vi "Run_Core.vi"(0 "Message Popup in":refnum<class "Array Functions.lvclass">, 11 "error in (no error)":errorcluster) -> (4 "Message Popup out":refnum<class "Array Functions.lvclass">, 6 "Return":variant, 15 "error out":errorcluster)   [LabVIEW 2019, in "Array Functions.lvclass"]
uses:
  Array Functions.lvclass
  C:/Users/Patrick/Documents/GitHub/LabVIEW-Script-Language/source code/LSL components/functions/functionsbase/functionbase.lvclass
  Array Functions.lvclass/Array Functions.ctl
  functionsbase/functionbase.lvclass/functionbase.ctl
  functionsbase/properties/Read RT Variables.vi
  functionsbase/properties/Read Indent#.vi
  data types/Variant to Data/Var to Numeric.vi
  data types/Variant to Data/Var to Boolean.vi
  variables/RT Variables/RT Variables.lvclass
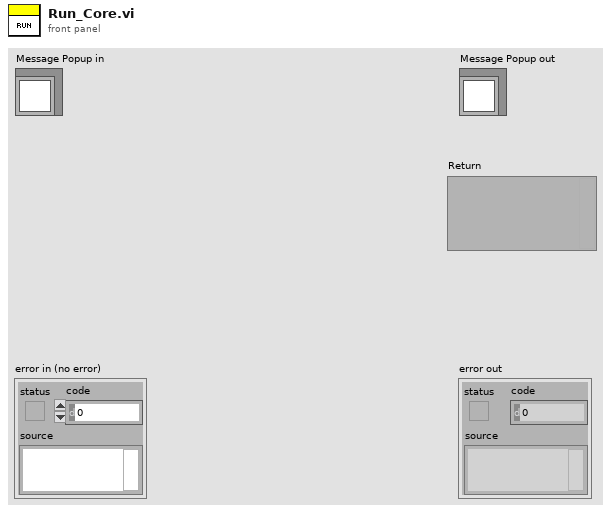
[diagram p1: front panel]
types:
  T1 = typedef "Array Functions.lvclass/Function List.ctl" = enum16{"Array Size", "Index Array", "Replace Subset", "Insert Into Array", "Delete From Array", "Initialize 1D Array", "Initialize 2D Array", "Build Array", "Array Subset", "Max in Array", "Min in Array", "Sort 1D Array", "Search 1D Aray", "Reverse 1D Array", "Slice by start stop", "Slice by start stop step", "range by start stop", "range by start stop step"}
  T2 = typedef "Datatype.ctl" = enum16{"Null", "Numeric", "String", "Bool", "Numeric 1D", "String 1D", "Bool 1D", "Numeric 2D", "String 2D", "Bool 2D", "Variant"}
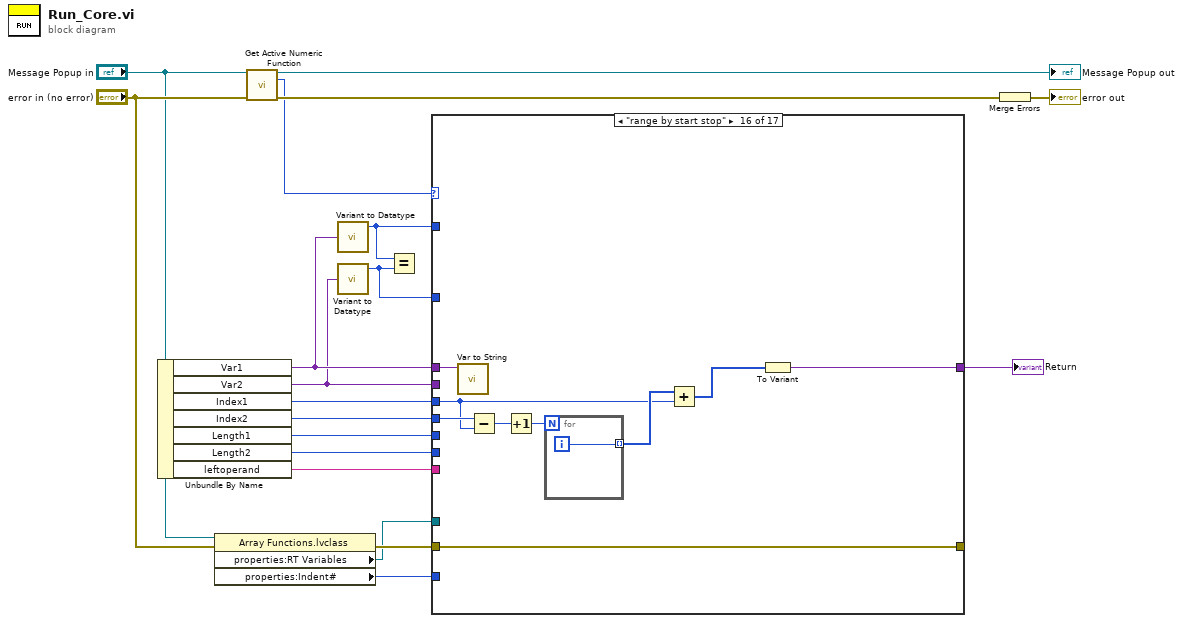
[diagram p0: block diagram]
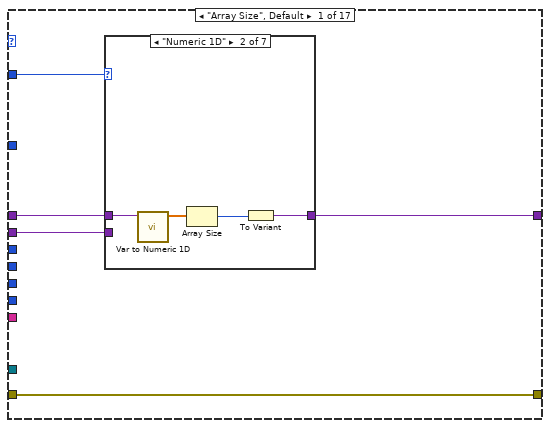
[diagram p2: hidden frame]
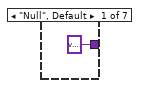
[diagram p3: hidden frame]
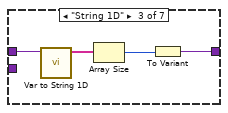
[diagram p4: hidden frame]
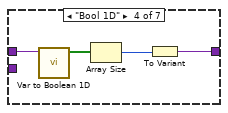
[diagram p5: hidden frame]
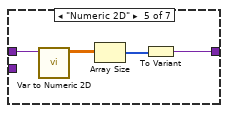
[diagram p6: hidden frame]
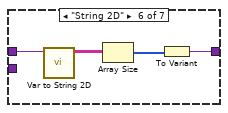
[diagram p7: hidden frame]
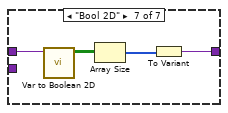
[diagram p8: hidden frame]
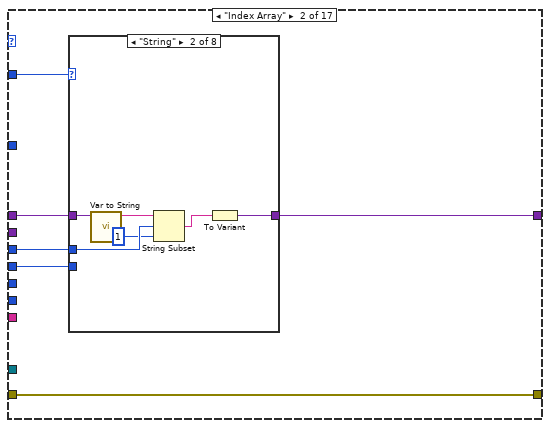
[diagram p9: hidden frame]
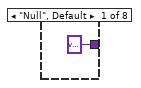
[diagram p10: hidden frame]
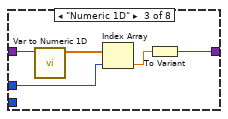
[diagram p11: hidden frame]
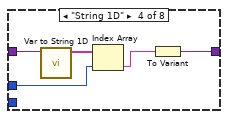
[diagram p12: hidden frame]
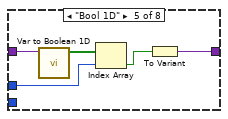
[diagram p13: hidden frame]
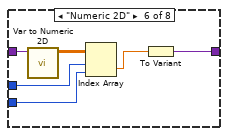
[diagram p14: hidden frame]
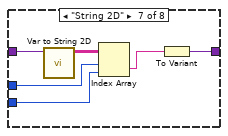
[diagram p15: hidden frame]
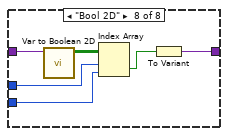
[diagram p16: hidden frame]
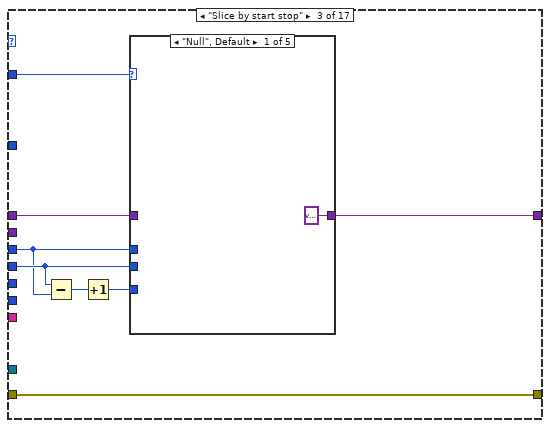
[diagram p17: hidden frame]
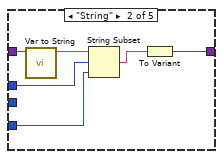
[diagram p18: hidden frame]
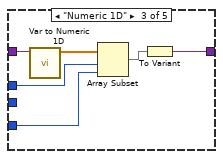
[diagram p19: hidden frame]
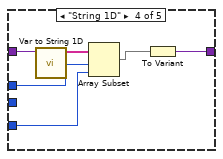
[diagram p20: hidden frame]
diagram:
  n1 = Unbundle By Name("Message Popup in") -> ("Var1"=w16:variant, "Var2"=w11:variant, "Index1"=w13:i32, "Index2"=w12:i32, "Length1"=w9:i32, "Length2"=w8:i32, "leftoperand"=w3:string)
  n2 = property class="Array Functions.lvclass"(reference="Message Popup in", error in="error in (no error)") -> (error out=w6:errorcluster, "properties:RT Variables"=w4:refnum<class "RT Variables.lvclass">, "properties:Indent#"=w2:i64)  [unwired: 1 out]
  n3 = call "Get Active Numeric Function.vi"("Numeric Functions in"="Message Popup in", "error in (no error)"="error in (no error)") -> ("Numeric Functions out"=→"Message Popup out":refnum<class "Array Functions.lvclass">, "Function"=w17:T1, "error out"=w18:errorcluster)  [unwired: 11 in]
  n4 = call "Variant to Datatype.vi"("Variant"=w16) -> ("Datatype"=w15:T2)  [unwired: 2 in, 2 out]
  n5 = call "Variant to Datatype.vi"("Variant"=w11) -> ("Datatype"=w10:T2)  [unwired: 2 in, 2 out]
  n6 = Equal?(x=w15, y=w10) -> ()  [unwired: 1 out]
  n7 = case shown="\"range by start stop\"" w17 {
    tunnel: w16 -> [w24 w55 w103 _ _ _ w319 w348 _ w493 w540 w568 _ w619 _ w671 w684]
    tunnel: w11 -> [w23 _ _ w140 w214 w289 _ _ w379 _ _ _ _ w617 _ _ _]
    tunnel: w15 -> [w22 w52 w101 _ _ _ w320 w345 _ w494 w541 w566 _ w618 _ _ _]
    tunnel: [w21 w54 w102 w131 w205 w278 w311 w338 w371 w490 w539 w567 w595 w615 w644 w670 w683] -> w14
    tunnel: w13 -> [_ w53 w98 w139 w213 w288 _ _ w378 w492 _ _ _ w616 _ w664 w679]
    tunnel: w12 -> [_ w51 w99 _ _ _ _ _ _ w489 _ _ _ _ _ w668 w681]
    tunnel: w10 -> [_ _ _ w141 w215 w290 _ _ w380 _ _ _ _ _ _ _ _]
    tunnel: w9 -> [_ _ _ _ _ w287 w318 w347 _ w491 _ _ _ _ _ _ w675]
    tunnel: w8 -> [_ _ _ _ _ _ _ w346 _ w488 _ _ _ _ _ _ _]
    tunnel: w6 -> [w20 w50 w100 w136 w210 w284 w317 w343 w375 w487 w538 w565 w599 w614 w648 w669 w682]
    tunnel: w4 -> [_ _ _ w135 w209 w281 w316 w342 w373 _ _ _ w598 _ w647 _ _]
    tunnel: w3 -> [_ _ _ w134 w206 w280 w312 w341 w372 _ _ _ w596 _ w645 _ _]
    tunnel: w2 -> [_ _ _ w132 w207 w282 w313 w339 w370 _ _ _ w597 _ w646 _ _]
    tunnel: [w20 w50 w100 w133 w208 w283 w310 w337 w374 w487 w538 w565 w594 w614 w643 w669 w682] -> _
    frame "Array Size", Default {
      n8 = case shown="\"Numeric 1D\"" w22 {
        tunnel: w24 -> [_ w29 w33 w37 w41 w45 w49]
        tunnel: w23 -> [_ _ _ _ _ _ _]
        tunnel: [variant ("Variant") w26 w30 w34 w38 w42 w46] -> w21
        frame "Null", Default {
        }
        frame "Numeric 1D" {
          n9 = call "Var to Numeric 1D.vi"("Variant"=w29) -> ("Numeric Array"=w28:dbl[])  [unwired: 10 in]
          n10 = Array Size(array=w28) -> (size(s)=w27:i32)
          n11 = To Variant(anything=w27) -> (Variant=w26:variant)
        }
        frame "String 1D" {
          n12 = call "Var to String 1D.vi"("Variant"=w33) -> ("String 1D"=w31:string[])  [unwired: 10 in]
          n13 = Array Size(array=w31) -> (size(s)=w32:i32)
          n14 = To Variant(anything=w32) -> (Variant=w30:variant)
        }
        frame "Bool 1D" {
          n15 = call "Var to Boolean 1D.vi"("Variant"=w37) -> ("Bool 1D"=w35:bool[])  [unwired: 10 in]
          n16 = Array Size(array=w35) -> (size(s)=w36:i32)
          n17 = To Variant(anything=w36) -> (Variant=w34:variant)
        }
        frame "Numeric 2D" {
          n18 = call "Var to Numeric 2D.vi"("Variant"=w41) -> ("Numeric Array"=w39:dbl[][])  [unwired: 10 in]
          n19 = Array Size(array=w39) -> (size(s)=w40:i32[])
          n20 = To Variant(anything=w40) -> (Variant=w38:variant)
        }
        frame "String 2D" {
          n21 = call "Var to String 2D.vi"("Variant"=w45) -> ("String 2D"=w43:string[][])  [unwired: 10 in]
          n22 = Array Size(array=w43) -> (size(s)=w44:i32[])
          n23 = To Variant(anything=w44) -> (Variant=w42:variant)
        }
        frame "Bool 2D" {
          n24 = call "Var to Boolean 2D.vi"("Variant"=w49) -> ("Bool 2D"=w47:bool[][])  [unwired: 10 in]
          n25 = Array Size(array=w47) -> (size(s)=w48:i32[])
          n26 = To Variant(anything=w48) -> (Variant=w46:variant)
        }
      }
    }
    frame "Index Array" {
      n27 = case shown="\"String\"" w52 {
        tunnel: w55 -> [_ w61 w67 w72 w77 w83 w89 w95]
        tunnel: [variant ("Variant") w62 w66 w71 w76 w82 w88 w94] -> w54
        tunnel: w53 -> [_ w59 w64 w68 w73 w79 w85 w91]
        tunnel: w51 -> [_ _ _ _ _ w78 w84 w90]
        frame "Null", Default {
        }
        frame "String" {
          n28 = call "Var to String.vi"("Variant"=w61) -> ("String"=w60:string)  [unwired: 10 in]
          n29 = String Subset(string=w60, offset (0)=w59, length (rest)=1 ("length (rest)")) -> (substring=w57:string)
          n30 = To Variant(anything=w57) -> (Variant=w62:variant)
        }
        frame "Numeric 1D" {
          n31 = call "Var to Numeric 1D.vi"("Variant"=w67) -> ("Numeric Array"=w65:dbl[])  [unwired: 10 in]
          n32 = Index Array(array=w65, index=w64) -> (element=w63:dbl)
          n33 = To Variant(anything=w63) -> (Variant=w66:variant)
        }
        frame "String 1D" {
          n34 = call "Var to String 1D.vi"("Variant"=w72) -> ("String 1D"=w70:string[])  [unwired: 10 in]
          n35 = Index Array(array=w70, index=w68) -> (element=w69:string)
          n36 = To Variant(anything=w69) -> (Variant=w71:variant)
        }
        frame "Bool 1D" {
          n37 = call "Var to Boolean 1D.vi"("Variant"=w77) -> ("Bool 1D"=w75:bool[])  [unwired: 10 in]
          n38 = Index Array(array=w75, index=w73) -> (element=w74:bool)
          n39 = To Variant(anything=w74) -> (Variant=w76:variant)
        }
        frame "Numeric 2D" {
          n40 = call "Var to Numeric 2D.vi"("Variant"=w83) -> ("Numeric Array"=w81:dbl[][])  [unwired: 10 in]
          n41 = Index Array(array=w81, index (row)=w79, index (col)=w78) -> (element=w80:dbl)
          n42 = To Variant(anything=w80) -> (Variant=w82:variant)
        }
        frame "String 2D" {
          n43 = call "Var to String 2D.vi"("Variant"=w89) -> ("String 2D"=w87:string[][])  [unwired: 10 in]
          n44 = Index Array(array=w87, index (row)=w85, index (col)=w84) -> (element=w86:string)
          n45 = To Variant(anything=w86) -> (Variant=w88:variant)
        }
        frame "Bool 2D" {
          n46 = call "Var to Boolean 2D.vi"("Variant"=w95) -> ("Bool 2D"=w93:bool[][])  [unwired: 10 in]
          n47 = Index Array(array=w93, index (row)=w91, index (col)=w90) -> (element=w92:bool)
          n48 = To Variant(anything=w92) -> (Variant=w94:variant)
        }
      }
    }
    frame "Slice by start stop" {
      n49 = Subtract(x=w99, y=w98) -> (x-y=w97:i32)
      n50 = Increment(x=w97) -> (x+1=w96:i32)
      n51 = case shown="\"Null\", Default" w101 {
        tunnel: w103 -> [_ w109 w116 w122 w128]
        tunnel: [variant ("Variant") w110 w115 w121 w127] -> w102
        tunnel: w98 -> [_ w106 w113 w118 w124]
        tunnel: w99 -> [_ _ _ _ _]
        tunnel: w96 -> [_ w105 w111 w117 w123]
        frame "Null", Default {
        }
        frame "String" {
          n52 = call "Var to String.vi"("Variant"=w109) -> ("String"=w108:string)  [unwired: 10 in]
          n53 = String Subset(string=w108, offset (0)=w106, length (rest)=w105) -> (substring=w107:string)
          n54 = To Variant(anything=w107) -> (Variant=w110:variant)
        }
        frame "Numeric 1D" {
          n55 = call "Var to Numeric 1D.vi"("Variant"=w116) -> ("Numeric Array"=w114:dbl[])  [unwired: 10 in]
          n56 = Array Subset(array=w114, index=w113, length=w111) -> (w112:dbl[])
          n57 = To Variant(anything=w112) -> (Variant=w115:variant)
        }
        frame "String 1D" {
          n58 = call "Var to String 1D.vi"("Variant"=w122) -> ("String 1D"=w120:string[])  [unwired: 10 in]
          n59 = Array Subset(array=w120, index=w118, length=w117) -> (w119:string[])
          n60 = To Variant(anything=w119) -> (Variant=w121:variant)
        }
        frame "Bool 1D" {
          n61 = call "Var to Boolean 1D.vi"("Variant"=w128) -> ("Bool 1D"=w126:bool[])  [unwired: 10 in]
          n62 = Array Subset(array=w126, index=w124, length=w123) -> (w125:bool[])
          n63 = To Variant(anything=w125) -> (Variant=w127:variant)
        }
      }
    }
    frame "Replace Subset" {
      n64 = call-dynamic "Retrieve RTV [by name].vi"("RT Variables in"=w135, "RTV name"=w134, "error in (no error)"=w136) -> ("RT Variables out"=w138:refnum<class "RT Variables.lvclass">, "Data"=w129:variant, "error out"=w137:errorcluster)  [unwired: 8 in, 2 out]
      n65 = call "Variant to Datatype.vi"("Variant"=w129) -> ("Datatype"=w130:T2)  [unwired: 2 in, 2 out]
      n66 = case shown="\"String 1D\"" w130 {
        tunnel: w129 -> [_ w147 w167 w187 _ _ _]
        tunnel: [variant ("Variant") w146 w163 w184 _ _ _] -> w131
        tunnel: w139 -> [_ w143 w164 w185 _ _ _]
        tunnel: w141 -> [_ w145 w166 w183 _ _ _]
        tunnel: w140 -> [_ w144 w165 w186 _ _ _]
        frame "Null", Default {
        }
        frame "Numeric 1D" {
          n67 = case shown="\"Numeric\"" w145 {
            tunnel: w147 -> [w151 w161 _]
            tunnel: [w150 w160 variant ("Variant")] -> w146
            tunnel: w144 -> [w149 w157 _]
            tunnel: w143 -> [w148 w156 _]
            frame "Numeric 1D" {
              n68 = call-poly "V2D_Poly.vi"("Variant"=w149) -> ("Numeric Array"=w152:dbl[])  [unwired: 10 in]
              n69 = call "Var to Numeric 1D.vi"("Variant"=w151) -> ("Numeric Array"=w154:dbl[])  [unwired: 10 in]
              n70 = Replace Array Subset(array=w154, new element=w152, index=w148) -> (w153:dbl[])
              n71 = To Variant(anything=w153) -> (Variant=w150:variant)
            }
            frame "Numeric" {
              n72 = call-poly "V2D_Poly.vi"("Variant"=w157) -> ("Numeric"=w155:dbl)  [unwired: 10 in]
              n73 = call "Var to Numeric 1D.vi"("Variant"=w161) -> ("Numeric Array"=w159:dbl[])  [unwired: 10 in]
              n74 = Replace Array Subset(array=w159, new element=w155, index=w156) -> (w158:dbl[])
              n75 = To Variant(anything=w158) -> (Variant=w160:variant)
            }
            frame Default {
            }
          }
        }
        frame "String 1D" {
          n76 = case shown="\"String 1D\"" w166 {
            tunnel: w167 -> [w171 w178 _]
            tunnel: [w172 w181 variant ("Variant")] -> w163
            tunnel: w165 -> [w169 w176 _]
            tunnel: w164 -> [w168 w175 _]
            frame "String 1D" {
              n77 = call-poly "V2D_Poly.vi"("Variant"=w171) -> ("String 1D"=w170:string[])  [unwired: 10 in]
              n78 = call-poly "V2D_Poly.vi"("Variant"=w169) -> ("String 1D"=w173:string[])  [unwired: 10 in]
              n79 = Replace Array Subset(array=w170, new element=w173, index=w168) -> (w174:string[])
              n80 = To Variant(anything=w174) -> (Variant=w172:variant)
            }
            frame "String" {
              n81 = call-poly "V2D_Poly.vi"("Variant"=w178) -> ("String 1D"=w177:string[])  [unwired: 10 in]
              n82 = call-poly "V2D_Poly.vi"("Variant"=w176) -> ("String"=w179:string)  [unwired: 10 in]
              n83 = Replace Array Subset(array=w177, new element=w179, index=w175) -> (w180:string[])
              n84 = To Variant(anything=w180) -> (Variant=w181:variant)
            }
            frame Default {
            }
          }
        }
        frame "Bool 1D" {
          n85 = case shown="\"Bool 1D\"" w183 {
            tunnel: w187 -> [w191 w198 _]
            tunnel: [w192 w201 variant ("Variant")] -> w184
            tunnel: w186 -> [w189 w196 _]
            tunnel: w185 -> [w188 w195 _]
            frame "Bool 1D" {
              n86 = call-poly "V2D_Poly.vi"("Variant"=w191) -> ("Bool 1D"=w190:bool[])  [unwired: 10 in]
              n87 = call-poly "V2D_Poly.vi"("Variant"=w189) -> ("Bool 1D"=w193:bool[])  [unwired: 10 in]
              n88 = Replace Array Subset(array=w190, new element=w193, index=w188) -> (w194:bool[])
              n89 = To Variant(anything=w194) -> (Variant=w192:variant)
            }
            frame "Bool" {
              n90 = call-poly "V2D_Poly.vi"("Variant"=w198) -> ("Bool 1D"=w197:bool[])  [unwired: 10 in]
              n91 = call-poly "V2D_Poly.vi"("Variant"=w196) -> ("Boolean"=w199:bool)  [unwired: 10 in]
              n92 = Replace Array Subset(array=w197, new element=w199, index=w195) -> (w200:bool[])
              n93 = To Variant(anything=w200) -> (Variant=w201:variant)
            }
            frame Default {
            }
          }
        }
        frame "Numeric 2D" {
        }
        frame "String 2D" {
        }
        frame "Bool 2D" {
        }
      }
      n94 = call-dynamic "Add RTV.vi"("RT Variables in"=w138, "RTV name"=w134, "Data"=w131, "Scope"=w132, "error in (no error)"=w137) -> ("error out"=w133:errorcluster)  [unwired: 9 in, 1 out]
    }
    frame "Insert Into Array" {
      n95 = call-dynamic "Retrieve RTV [by name].vi"("RT Variables in"=w209, "RTV name"=w206, "error in (no error)"=w210) -> ("RT Variables out"=w212:refnum<class "RT Variables.lvclass">, "Data"=w203:variant, "error out"=w211:errorcluster)  [unwired: 8 in, 2 out]
      n96 = call "Variant to Datatype.vi"("Variant"=w203) -> ("Datatype"=w204:T2)  [unwired: 2 in, 2 out]
      n97 = case shown="\"Numeric 1D\"" w204 {
        tunnel: w203 -> [_ w221 w241 w261 _ _ _]
        tunnel: [variant ("Variant") w220 w237 w258 _ _ _] -> w205
        tunnel: w213 -> [_ w217 w238 w259 _ _ _]
        tunnel: w215 -> [_ w219 w240 w257 _ _ _]
        tunnel: w214 -> [_ w218 w239 w260 _ _ _]
        frame "Null", Default {
        }
        frame "Numeric 1D" {
          n98 = case shown="\"Numeric\"" w219 {
            tunnel: w221 -> [w225 w235 _]
            tunnel: [w224 w234 variant ("Variant")] -> w220
            tunnel: w218 -> [w223 w231 _]
            tunnel: w217 -> [w222 w230 _]
            frame "Numeric 1D" {
              n99 = call-poly "V2D_Poly.vi"("Variant"=w223) -> ("Numeric Array"=w226:dbl[])  [unwired: 10 in]
              n100 = call "Var to Numeric 1D.vi"("Variant"=w225) -> ("Numeric Array"=w228:dbl[])  [unwired: 10 in]
              n101 = Insert Into Array(array=w228, index=w222, new element=w226) -> (w227:dbl[])
              n102 = To Variant(anything=w227) -> (Variant=w224:variant)
            }
            frame "Numeric" {
              n103 = call-poly "V2D_Poly.vi"("Variant"=w231) -> ("Numeric"=w229:dbl)  [unwired: 10 in]
              n104 = call "Var to Numeric 1D.vi"("Variant"=w235) -> ("Numeric Array"=w233:dbl[])  [unwired: 10 in]
              n105 = Insert Into Array(array=w233, index=w230, new element=w229) -> (w232:dbl[])
              n106 = To Variant(anything=w232) -> (Variant=w234:variant)
            }
            frame Default {
            }
          }
        }
        frame "String 1D" {
          n107 = case shown="\"String\"" w240 {
            tunnel: w241 -> [w245 w252 _]
            tunnel: [w246 w255 variant ("Variant")] -> w237
            tunnel: w239 -> [w243 w250 _]
            tunnel: w238 -> [w242 w249 _]
            frame "String 1D" {
              n108 = call-poly "V2D_Poly.vi"("Variant"=w245) -> ("String 1D"=w244:string[])  [unwired: 10 in]
              n109 = call-poly "V2D_Poly.vi"("Variant"=w243) -> ("String 1D"=w247:string[])  [unwired: 10 in]
              n110 = Insert Into Array(array=w244, index=w242, new element=w247) -> (w248:string[])
              n111 = To Variant(anything=w248) -> (Variant=w246:variant)
            }
            frame "String" {
              n112 = call-poly "V2D_Poly.vi"("Variant"=w252) -> ("String 1D"=w251:string[])  [unwired: 10 in]
              n113 = call-poly "V2D_Poly.vi"("Variant"=w250) -> ("String"=w253:string)  [unwired: 10 in]
              n114 = Insert Into Array(array=w251, index=w249, new element=w253) -> (w254:string[])
              n115 = To Variant(anything=w254) -> (Variant=w255:variant)
            }
            frame Default {
            }
          }
        }
        frame "Bool 1D" {
          n116 = case shown="\"Bool 1D\"" w257 {
            tunnel: w261 -> [w265 w272 _]
            tunnel: [w266 w275 variant ("Variant")] -> w258
            tunnel: w260 -> [w263 w270 _]
            tunnel: w259 -> [w262 w269 _]
            frame "Bool 1D" {
              n117 = call-poly "V2D_Poly.vi"("Variant"=w265) -> ("Bool 1D"=w264:bool[])  [unwired: 10 in]
              n118 = call-poly "V2D_Poly.vi"("Variant"=w263) -> ("Bool 1D"=w267:bool[])  [unwired: 10 in]
              n119 = Insert Into Array(array=w264, index=w262, new element=w267) -> (w268:bool[])
              n120 = To Variant(anything=w268) -> (Variant=w266:variant)
            }
            frame "Bool" {
              n121 = call-poly "V2D_Poly.vi"("Variant"=w272) -> ("Bool 1D"=w271:bool[])  [unwired: 10 in]
              n122 = call-poly "V2D_Poly.vi"("Variant"=w270) -> ("Boolean"=w273:bool)  [unwired: 10 in]
              n123 = Insert Into Array(array=w271, index=w269, new element=w273) -> (w274:bool[])
              n124 = To Variant(anything=w274) -> (Variant=w275:variant)
            }
            frame Default {
            }
          }
        }
        frame "Numeric 2D" {
        }
        frame "String 2D" {
        }
        frame "Bool 2D" {
        }
      }
      n125 = call-dynamic "Add RTV.vi"("RT Variables in"=w212, "RTV name"=w206, "Data"=w205, "Scope"=w207, "error in (no error)"=w211) -> ("error out"=w208:errorcluster)  [unwired: 9 in, 1 out]
    }
    frame "Delete From Array" {
      n126 = call-dynamic "Retrieve RTV [by name].vi"("RT Variables in"=w281, "RTV name"=w280, "error in (no error)"=w284) -> ("RT Variables out"=w286:refnum<class "RT Variables.lvclass">, "Data"=w277:variant, "error out"=w285:errorcluster)  [unwired: 8 in, 2 out]
      n127 = call "Variant to Datatype.vi"("Variant"=w277) -> ("Datatype"=w279:T2)  [unwired: 2 in, 2 out]
      n128 = case shown="\"String 1D\"" w279 {
        tunnel: w277 -> [_ w297 w303 w309 _ _ _]
        tunnel: [variant ("Variant") w296 w302 w308 _ _ _] -> w278
        tunnel: w288 -> [_ w293 w299 w305 _ _ _]
        tunnel: w290 -> [_ _ _ _ _ _ _]
        tunnel: w289 -> [_ _ _ _ _ _ _]
        tunnel: w287 -> [_ w292 w298 w304 _ _ _]
        frame "Null", Default {
        }
        frame "Numeric 1D" {
          n129 = call "Var to Numeric 1D.vi"("Variant"=w297) -> ("Numeric Array"=w295:dbl[])  [unwired: 10 in]
          n130 = Delete From Array(array=w295, length=w292, index=w293) -> (array with subset deleted=w294:dbl[])  [unwired: 1 out]
          n131 = To Variant(anything=w294) -> (Variant=w296:variant)
        }
        frame "String 1D" {
          n132 = call-poly "V2D_Poly.vi"("Variant"=w303) -> ("String 1D"=w300:string[])  [unwired: 10 in]
          n133 = Delete From Array(array=w300, length=w298, index=w299) -> (array with subset deleted=w301:string[])  [unwired: 1 out]
          n134 = To Variant(anything=w301) -> (Variant=w302:variant)
        }
        frame "Bool 1D" {
          n135 = call-poly "V2D_Poly.vi"("Variant"=w309) -> ("Bool 1D"=w306:bool[])  [unwired: 10 in]
          n136 = Delete From Array(array=w306, length=w304, index=w305) -> (array with subset deleted=w307:bool[])  [unwired: 1 out]
          n137 = To Variant(anything=w307) -> (Variant=w308:variant)
        }
        frame "Numeric 2D" {
        }
        frame "String 2D" {
        }
        frame "Bool 2D" {
        }
      }
      n138 = call-dynamic "Add RTV.vi"("RT Variables in"=w286, "RTV name"=w280, "Data"=w278, "Scope"=w282, "error in (no error)"=w285) -> ("error out"=w283:errorcluster)  [unwired: 9 in, 1 out]
    }
    frame "Initialize 1D Array" {
      n139 = call-dynamic "Retrieve RTV [by name].vi"("RT Variables in"=w316, "RTV name"=w312, "error in (no error)"=w317) -> ("RT Variables out"=w314:refnum<class "RT Variables.lvclass">, "error out"=w315:errorcluster)  [unwired: 8 in, 3 out]
      n140 = case shown="\"Numeric\"" w320 {
        tunnel: w319 -> [_ w324 w329 w336]
        tunnel: w318 -> [_ w322 w327 w334]
        tunnel: [variant ("Variant") w323 w328 w332] -> w311
        frame "Null", Default {
        }
        frame "Numeric" {
          n141 = call-poly "V2D_Poly.vi"("Variant"=w324) -> ("Numeric"=w326:dbl)  [unwired: 10 in]
          n142 = Initialize Array(w326, w322) -> (w325:dbl[])
          n143 = To Variant(anything=w325) -> (Variant=w323:variant)
        }
        frame "String" {
          n144 = call-poly "V2D_Poly.vi"("Variant"=w329) -> ("String"=w331:string)  [unwired: 10 in]
          n145 = Initialize Array(w331, w327) -> (w330:string[])
          n146 = To Variant(anything=w330) -> (Variant=w328:variant)
        }
        frame "Bool" {
          n147 = call-poly "V2D_Poly.vi"("Variant"=w336) -> ("Boolean"=w335:bool)  [unwired: 10 in]
          n148 = Initialize Array(w335, w334) -> (w333:bool[])
          n149 = To Variant(anything=w333) -> (Variant=w332:variant)
        }
      }
      n150 = call-dynamic "Add RTV.vi"("RT Variables in"=w314, "RTV name"=w312, "Data"=w311, "Scope"=w313, "error in (no error)"=w315) -> ("error out"=w310:errorcluster)  [unwired: 9 in, 1 out]
    }
    frame "Initialize 2D Array" {
      n151 = call-dynamic "Retrieve RTV [by name].vi"("RT Variables in"=w342, "RTV name"=w341, "error in (no error)"=w343) -> ("RT Variables out"=w344:refnum<class "RT Variables.lvclass">, "error out"=w340:errorcluster)  [unwired: 8 in, 3 out]
      n152 = case shown="\"String\"" w345 {
        tunnel: w348 -> [_ w353 w359 w367]
        tunnel: w347 -> [_ w351 w357 w365]
        tunnel: [variant ("Variant") w352 w358 w363] -> w338
        tunnel: w346 -> [_ w350 w356 w362]
        frame "Null", Default {
        }
        frame "Numeric" {
          n153 = call-poly "V2D_Poly.vi"("Variant"=w353) -> ("Numeric"=w355:dbl)  [unwired: 10 in]
          n154 = Initialize Array(w355, w351, w350) -> (w354:dbl[][])
          n155 = To Variant(anything=w354) -> (Variant=w352:variant)
        }
        frame "String" {
          n156 = call-poly "V2D_Poly.vi"("Variant"=w359) -> ("String"=w361:string)  [unwired: 10 in]
          n157 = Initialize Array(w361, w357, w356) -> (w360:string[][])
          n158 = To Variant(anything=w360) -> (Variant=w358:variant)
        }
        frame "Bool" {
          n159 = call-poly "V2D_Poly.vi"("Variant"=w367) -> ("Boolean"=w366:bool)  [unwired: 10 in]
          n160 = Initialize Array(w366, w365, w362) -> (w364:bool[][])
          n161 = To Variant(anything=w364) -> (Variant=w363:variant)
        }
      }
      n162 = call-dynamic "Add RTV.vi"("RT Variables in"=w344, "RTV name"=w341, "Data"=w338, "Scope"=w339, "error in (no error)"=w340) -> ("error out"=w337:errorcluster)  [unwired: 9 in, 1 out]
    }
    frame "Build Array" {
      # "append"
      n163 = call-dynamic "Retrieve RTV [by name].vi"("RT Variables in"=w373, "RTV name"=w372, "error in (no error)"=w375) -> ("RT Variables out"=w377:refnum<class "RT Variables.lvclass">, "Data"=w368:variant, "error out"=w376:errorcluster)  [unwired: 8 in, 2 out]
      n164 = call "Variant to Datatype.vi"("Variant"=w368) -> ("Datatype"=w369:T2)  [unwired: 2 in, 2 out]
      n165 = case shown="\"String 1D\"" w369 {
        tunnel: w368 -> [_ w386 w404 w422 w439 w456 w473]
        tunnel: [variant ("Variant") w385 w400 w419 w437 w453 w470] -> w371
        tunnel: w378 -> [_ w382 w401 w420 _ _ _]
        tunnel: w380 -> [_ w384 w403 w418 w436 w454 w471]
        tunnel: w379 -> [_ w383 w402 w421 w438 w455 w472]
        frame "Null", Default {
        }
        frame "Numeric 1D" {
          n166 = case shown="Default" w384 {
            tunnel: w386 -> [w389 w398 _]
            tunnel: [w388 w397 variant ("Variant")] -> w385
            tunnel: w383 -> [w387 w394 _]
            tunnel: w382 -> [_ _ _]
            frame "Numeric 1D" {
              n167 = call-poly "V2D_Poly.vi"("Variant"=w387) -> ("Numeric Array"=w390:dbl[])  [unwired: 10 in]
              n168 = call "Var to Numeric 1D.vi"("Variant"=w389) -> ("Numeric Array"=w392:dbl[])  [unwired: 10 in]
              n169 = Build Array (concatenate)(w392, w390) -> (w391:dbl[])
              n170 = To Variant(anything=w391) -> (Variant=w388:variant)
            }
            frame "Numeric" {
              n171 = call-poly "V2D_Poly.vi"("Variant"=w394) -> ("Numeric"=w393:dbl)  [unwired: 10 in]
              n172 = call "Var to Numeric 1D.vi"("Variant"=w398) -> ("Numeric Array"=w396:dbl[])  [unwired: 10 in]
              n173 = Build Array (concatenate)(w396, w393) -> (w395:dbl[])
              n174 = To Variant(anything=w395) -> (Variant=w397:variant)
            }
            frame Default {
            }
          }
        }
        frame "String 1D" {
          n175 = case shown="Default" w403 {
            tunnel: w404 -> [w407 w413 _]
            tunnel: [w408 w416 variant ("Variant")] -> w400
            tunnel: w402 -> [w405 w411 _]
            tunnel: w401 -> [_ _ _]
            frame "String 1D" {
              n176 = call-poly "V2D_Poly.vi"("Variant"=w407) -> ("String 1D"=w406:string[])  [unwired: 10 in]
              n177 = call-poly "V2D_Poly.vi"("Variant"=w405) -> ("String 1D"=w409:string[])  [unwired: 10 in]
              n178 = Build Array (concatenate)(w406, w409) -> (w410:string[])
              n179 = To Variant(anything=w410) -> (Variant=w408:variant)
            }
            frame "String" {
              n180 = call-poly "V2D_Poly.vi"("Variant"=w413) -> ("String 1D"=w412:string[])  [unwired: 10 in]
              n181 = call-poly "V2D_Poly.vi"("Variant"=w411) -> ("String"=w414:string)  [unwired: 10 in]
              n182 = Build Array (concatenate)(w412, w414) -> (w415:string[])
              n183 = To Variant(anything=w415) -> (Variant=w416:variant)
            }
            frame Default {
            }
          }
        }
        frame "Bool 1D" {
          n184 = case shown="\"Bool\"" w418 {
            tunnel: w422 -> [w425 w431 _]
            tunnel: [w426 w434 variant ("Variant")] -> w419
            tunnel: w421 -> [w423 w429 _]
            tunnel: w420 -> [_ _ _]
            frame "Bool 1D" {
              n185 = call-poly "V2D_Poly.vi"("Variant"=w425) -> ("Bool 1D"=w424:bool[])  [unwired: 10 in]
              n186 = call-poly "V2D_Poly.vi"("Variant"=w423) -> ("Bool 1D"=w427:bool[])  [unwired: 10 in]
              n187 = Build Array (concatenate)(w424, w427) -> (w428:bool[])
              n188 = To Variant(anything=w428) -> (Variant=w426:variant)
            }
            frame "Bool" {
              n189 = call-poly "V2D_Poly.vi"("Variant"=w431) -> ("Bool 1D"=w430:bool[])  [unwired: 10 in]
              n190 = call-poly "V2D_Poly.vi"("Variant"=w429) -> ("Boolean"=w432:bool)  [unwired: 10 in]
              n191 = Build Array (concatenate)(w430, w432) -> (w433:bool[])
              n192 = To Variant(anything=w433) -> (Variant=w434:variant)
            }
            frame Default {
            }
          }
        }
        frame "Numeric 2D" {
          n193 = case shown="\"Numeric 2D\"" w436 {
            tunnel: w439 -> [w441 w447 _]
            tunnel: [w443 w451 variant ("Variant")] -> w437
            tunnel: w438 -> [w442 w449 _]
            frame "Numeric 1D" {
              n194 = call-poly "V2D_Poly.vi"("Variant"=w442) -> ("Numeric Array"=w444:dbl[])  [unwired: 10 in]
              n195 = call-poly "V2D_Poly.vi"("Variant"=w441) -> ("Numeric Array"=w440:dbl[][])  [unwired: 10 in]
              n196 = Build Array (concatenate)(w440, w444) -> (w445:dbl[][])
              n197 = To Variant(anything=w445) -> (Variant=w443:variant)
            }
            frame "Numeric 2D" {
              n198 = call-poly "V2D_Poly.vi"("Variant"=w447) -> ("Numeric Array"=w446:dbl[][])  [unwired: 10 in]
              n199 = call-poly "V2D_Poly.vi"("Variant"=w449) -> ("Numeric Array"=w448:dbl[][])  [unwired: 10 in]
              n200 = Build Array (concatenate)(w446, w448) -> (w450:dbl[][])
              n201 = To Variant(anything=w450) -> (Variant=w451:variant)
            }
            frame Default {
            }
          }
        }
        frame "String 2D" {
          n202 = case shown="\"String 2D\"" w454 {
            tunnel: w456 -> [w459 w465 _]
            tunnel: [w460 w468 variant ("Variant")] -> w453
            tunnel: w455 -> [w457 w463 _]
            frame "String 1D" {
              n203 = call-poly "V2D_Poly.vi"("Variant"=w459) -> ("String 2D"=w458:string[][])  [unwired: 10 in]
              n204 = call-poly "V2D_Poly.vi"("Variant"=w457) -> ("String 1D"=w461:string[])  [unwired: 10 in]
              n205 = Build Array (concatenate)(w458, w461) -> (w462:string[][])
              n206 = To Variant(anything=w462) -> (Variant=w460:variant)
            }
            frame "String 2D" {
              n207 = call-poly "V2D_Poly.vi"("Variant"=w465) -> ("String 2D"=w464:string[][])  [unwired: 10 in]
              n208 = call-poly "V2D_Poly.vi"("Variant"=w463) -> ("String 2D"=w466:string[][])  [unwired: 10 in]
              n209 = Build Array (concatenate)(w464, w466) -> (w467:string[][])
              n210 = To Variant(anything=w467) -> (Variant=w468:variant)
            }
            frame Default {
            }
          }
        }
        frame "Bool 2D" {
          n211 = case shown="Default" w471 {
            tunnel: w473 -> [w476 w482 _]
            tunnel: [w477 w485 variant ("Variant")] -> w470
            tunnel: w472 -> [w474 w480 _]
            frame "Bool 1D" {
              n212 = call-poly "V2D_Poly.vi"("Variant"=w476) -> ("Bool 2D"=w475:bool[][])  [unwired: 10 in]
              n213 = call-poly "V2D_Poly.vi"("Variant"=w474) -> ("Bool 1D"=w478:bool[])  [unwired: 10 in]
              n214 = Build Array (concatenate)(w475, w478) -> (w479:bool[][])
              n215 = To Variant(anything=w479) -> (Variant=w477:variant)
            }
            frame "Bool 2D" {
              n216 = call-poly "V2D_Poly.vi"("Variant"=w482) -> ("Bool 2D"=w481:bool[][])  [unwired: 10 in]
              n217 = call-poly "V2D_Poly.vi"("Variant"=w480) -> ("Bool 2D"=w483:bool[][])  [unwired: 10 in]
              n218 = Build Array (concatenate)(w481, w483) -> (w484:bool[][])
              n219 = To Variant(anything=w484) -> (Variant=w485:variant)
            }
            frame Default {
            }
          }
        }
      }
      n220 = call-dynamic "Add RTV.vi"("RT Variables in"=w377, "RTV name"=w372, "Data"=w371, "Scope"=w370, "error in (no error)"=w376) -> ("error out"=w374:errorcluster)  [unwired: 9 in, 1 out]
    }
    frame "Array Subset" {
      n221 = case shown="\"Bool 1D\"" w494 {
        tunnel: w493 -> [_ w501 w505 w512 w520 w528 w536]
        tunnel: w492 -> [_ w499 w503 w511 w518 w526 w534]
        tunnel: w491 -> [_ w498 w502 w510 w517 w525 w533]
        tunnel: [variant ("Variant") w496 w504 w508 w514 w522 w530] -> w490
        tunnel: w489 -> [_ _ _ _ w516 w524 w532]
        tunnel: w488 -> [_ _ _ _ w515 w523 w531]
        frame "Null", Default {
        }
        frame "Numeric 1D" {
          n222 = call-poly "V2D_Poly.vi"("Variant"=w501) -> ("Numeric Array"=w500:dbl[])  [unwired: 10 in]
          n223 = Array Subset(array=w500, index=w499, length=w498) -> (w497:dbl[])
          n224 = To Variant(anything=w497) -> (Variant=w496:variant)
        }
        frame "String 1D" {
          n225 = call-poly "V2D_Poly.vi"("Variant"=w505) -> ("String 1D"=w507:string[])  [unwired: 10 in]
          n226 = Array Subset(array=w507, index=w503, length=w502) -> (w506:string[])
          n227 = To Variant(anything=w506) -> (Variant=w504:variant)
        }
        frame "Bool 1D" {
          n228 = call-poly "V2D_Poly.vi"("Variant"=w512) -> ("Bool 1D"=w513:bool[])  [unwired: 10 in]
          n229 = Array Subset(array=w513, index=w511, length=w510) -> (w509:bool[])
          n230 = To Variant(anything=w509) -> (Variant=w508:variant)
        }
        frame "Numeric 2D" {
          n231 = call-poly "V2D_Poly.vi"("Variant"=w520) -> ("Numeric Array"=w521:dbl[][])  [unwired: 10 in]
          n232 = Array Subset(array=w521, index (row)=w518, length (row)=w517, index (col)=w516, length (col)=w515) -> (w519:dbl[][])
          n233 = To Variant(anything=w519) -> (Variant=w514:variant)
        }
        frame "String 2D" {
          n234 = call-poly "V2D_Poly.vi"("Variant"=w528) -> ("String 2D"=w529:string[][])  [unwired: 10 in]
          n235 = Array Subset(array=w529, index (row)=w526, length (row)=w525, index (col)=w524, length (col)=w523) -> (w527:string[][])
          n236 = To Variant(anything=w527) -> (Variant=w522:variant)
        }
        frame "Bool 2D" {
          n237 = call-poly "V2D_Poly.vi"("Variant"=w536) -> ("Bool 2D"=w537:bool[][])  [unwired: 10 in]
          n238 = Array Subset(array=w537, index (row)=w534, length (row)=w533, index (col)=w532, length (col)=w531) -> (w535:bool[][])
          n239 = To Variant(anything=w535) -> (Variant=w530:variant)
        }
      }
    }
    frame "Max in Array" {
      n240 = case shown="\"Numeric 2D\"" w541 {
        tunnel: w540 -> [_ _ _ _ w549 w551 _ w556 w560 _ _]
        tunnel: [variant ("Variant") variant ("Variant") variant ("Variant") variant ("Variant") w546 w550 variant ("Variant") w555 w559 variant ("Variant") variant ("Variant")] -> w539
        frame "Null", Default {
        }
        frame "Numeric" {
        }
        frame "String" {
        }
        frame "Bool" {
        }
        frame "Numeric 1D" {
          n241 = call-poly "V2D_Poly.vi"("Variant"=w549) -> ("Numeric Array"=w548:dbl[])  [unwired: 10 in]
          n242 = Array Max & Min(array=w548) -> (max value=w547:dbl)  [unwired: 3 out]
          n243 = To Variant(anything=w547) -> (Variant=w546:variant)
        }
        frame "String 1D" {
          n244 = call-poly "V2D_Poly.vi"("Variant"=w551) -> ("String 1D"=w553:string[])  [unwired: 10 in]
          n245 = Array Max & Min(array=w553) -> (max value=w552:string)  [unwired: 3 out]
          n246 = To Variant(anything=w552) -> (Variant=w550:variant)
        }
        frame "Bool 1D" {
        }
        frame "Numeric 2D" {
          n247 = call-poly "V2D_Poly.vi"("Variant"=w556) -> ("Numeric Array"=w558:dbl[][])  [unwired: 10 in]
          n248 = Array Max & Min(array=w558) -> (max value=w557:dbl)  [unwired: 3 out]
          n249 = To Variant(anything=w557) -> (Variant=w555:variant)
        }
        frame "String 2D" {
          n250 = call-poly "V2D_Poly.vi"("Variant"=w560) -> ("String 2D"=w562:string[][])  [unwired: 10 in]
          n251 = Array Max & Min(array=w562) -> (max value=w561:string)  [unwired: 3 out]
          n252 = To Variant(anything=w561) -> (Variant=w559:variant)
        }
        frame "Bool 2D" {
        }
        frame "Variant" {
        }
      }
    }
    frame "Min in Array" {
      n253 = case shown="\"String 1D\"" w566 {
        tunnel: w568 -> [_ _ _ _ w576 w579 _ w584 w588 _ _]
        tunnel: [variant ("Variant") variant ("Variant") variant ("Variant") variant ("Variant") w574 w578 variant ("Variant") w583 w587 variant ("Variant") variant ("Variant")] -> w567
        frame "Null", Default {
        }
        frame "Numeric" {
        }
        frame "String" {
        }
        frame "Bool" {
        }
        frame "Numeric 1D" {
          n254 = call-poly "V2D_Poly.vi"("Variant"=w576) -> ("Numeric Array"=w575:dbl[])  [unwired: 10 in]
          n255 = Array Max & Min(array=w575) -> (min value=w573:dbl)  [unwired: 3 out]
          n256 = To Variant(anything=w573) -> (Variant=w574:variant)
        }
        frame "String 1D" {
          n257 = call-poly "V2D_Poly.vi"("Variant"=w579) -> ("String 1D"=w580:string[])  [unwired: 10 in]
          n258 = Array Max & Min(array=w580) -> (min value=w577:string)  [unwired: 3 out]
          n259 = To Variant(anything=w577) -> (Variant=w578:variant)
        }
        frame "Bool 1D" {
        }
        frame "Numeric 2D" {
          n260 = call-poly "V2D_Poly.vi"("Variant"=w584) -> ("Numeric Array"=w585:dbl[][])  [unwired: 10 in]
          n261 = Array Max & Min(array=w585) -> (min value=w582:dbl)  [unwired: 3 out]
          n262 = To Variant(anything=w582) -> (Variant=w583:variant)
        }
        frame "String 2D" {
          n263 = call-poly "V2D_Poly.vi"("Variant"=w588) -> ("String 2D"=w589:string[][])  [unwired: 10 in]
          n264 = Array Max & Min(array=w589) -> (min value=w586:string)  [unwired: 3 out]
          n265 = To Variant(anything=w586) -> (Variant=w587:variant)
        }
        frame "Bool 2D" {
        }
        frame "Variant" {
        }
      }
    }
    frame "Sort 1D Array" {
      n266 = call-dynamic "Retrieve RTV [by name].vi"("RT Variables in"=w598, "RTV name"=w596, "error in (no error)"=w599) -> ("RT Variables out"=w601:refnum<class "RT Variables.lvclass">, "Data"=w592:variant, "error out"=w600:errorcluster)  [unwired: 8 in, 2 out]
      n267 = call "Variant to Datatype.vi"("Variant"=w592) -> ("Datatype"=w593:T2)  [unwired: 2 in, 2 out]
      n268 = case shown="\"Numeric 1D\"" w593 {
        tunnel: w592 -> [_ w605 w607 w611]
        tunnel: [_ w602 w606 w610] -> w595
        frame "Null", Default {
        }
        frame "Numeric 1D" {
          n269 = call-poly "V2D_Poly.vi"("Variant"=w605) -> ("Numeric Array"=w604:dbl[])  [unwired: 10 in]
          n270 = Sort 1D Array(array=w604) -> (sorted array=w603:dbl[])
          n271 = To Variant(anything=w603) -> (Variant=w602:variant)
        }
        frame "String 1D" {
          n272 = call-poly "V2D_Poly.vi"("Variant"=w607) -> ("String 1D"=w609:string[])  [unwired: 10 in]
          n273 = Sort 1D Array(array=w609) -> (sorted array=w608:string[])
          n274 = To Variant(anything=w608) -> (Variant=w606:variant)
        }
        frame "Bool 1D" {
          n275 = call-poly "V2D_Poly.vi"("Variant"=w611) -> ("Bool 1D"=w613:bool[])  [unwired: 10 in]
          n276 = Sort 1D Array(array=w613) -> (sorted array=w612:bool[])
          n277 = To Variant(anything=w612) -> (Variant=w610:variant)
        }
      }
      n278 = call-dynamic "Add RTV.vi"("RT Variables in"=w601, "RTV name"=w596, "Data"=w595, "Scope"=w597, "error in (no error)"=w600) -> ("error out"=w594:errorcluster)  [unwired: 9 in, 1 out]
    }
    frame "Search 1D Aray" {
      n279 = case shown="\"Numeric 1D\"" w618 {
        tunnel: w619 -> [_ w626 w633 w640]
        tunnel: [_ w624 w632 w639] -> w615
        tunnel: w617 -> [_ w622 w630 w636]
        tunnel: w616 -> [_ w620 w628 w634]
        frame "Null", Default {
        }
        frame "Numeric 1D" {
          n280 = call-poly "V2D_Poly.vi"("Variant"=w626) -> ("Numeric Array"=w623:dbl[])  [unwired: 10 in]
          n281 = call-poly "V2D_Poly.vi"("Variant"=w622) -> ("Numeric"=w621:dbl)  [unwired: 10 in]
          n282 = Search 1D Array(1D array=w623, element=w621, start index (0)=w620) -> (index of element=w625:i32)
          n283 = To Variant(anything=w625) -> (Variant=w624:variant)
        }
        frame "String 1D" {
          n284 = call-poly "V2D_Poly.vi"("Variant"=w633) -> ("String 1D"=w631:string[])  [unwired: 10 in]
          n285 = call-poly "V2D_Poly.vi"("Variant"=w630) -> ("String"=w629:string)  [unwired: 10 in]
          n286 = Search 1D Array(1D array=w631, element=w629, start index (0)=w628) -> (index of element=w627:i32)
          n287 = To Variant(anything=w627) -> (Variant=w632:variant)
        }
        frame "Bool 1D" {
          n288 = call-poly "V2D_Poly.vi"("Variant"=w640) -> ("Bool 1D"=w638:bool[])  [unwired: 10 in]
          n289 = call-poly "V2D_Poly.vi"("Variant"=w636) -> ("Boolean"=w635:bool)  [unwired: 10 in]
          n290 = Search 1D Array(1D array=w638, element=w635, start index (0)=w634) -> (index of element=w637:i32)
          n291 = To Variant(anything=w637) -> (Variant=w639:variant)
        }
      }
    }
    frame "Reverse 1D Array" {
      n292 = call-dynamic "Retrieve RTV [by name].vi"("RT Variables in"=w647, "RTV name"=w645, "error in (no error)"=w648) -> ("RT Variables out"=w650:refnum<class "RT Variables.lvclass">, "Data"=w641:variant, "error out"=w649:errorcluster)  [unwired: 8 in, 2 out]
      n293 = call "Variant to Datatype.vi"("Variant"=w641) -> ("Datatype"=w642:T2)  [unwired: 2 in, 2 out]
      n294 = case shown="\"Numeric 1D\"" w642 {
        tunnel: w641 -> [_ w654 w656 w660]
        tunnel: [_ w651 w655 w659] -> w644
        frame "Null", Default {
        }
        frame "Numeric 1D" {
          n295 = call-poly "V2D_Poly.vi"("Variant"=w654) -> ("Numeric Array"=w653:dbl[])  [unwired: 10 in]
          n296 = Reverse 1D Array(array=w653) -> (reversed array=w652:dbl[])
          n297 = To Variant(anything=w652) -> (Variant=w651:variant)
        }
        frame "String 1D" {
          n298 = call-poly "V2D_Poly.vi"("Variant"=w656) -> ("String 1D"=w658:string[])  [unwired: 10 in]
          n299 = Reverse 1D Array(array=w658) -> (reversed array=w657:string[])
          n300 = To Variant(anything=w657) -> (Variant=w655:variant)
        }
        frame "Bool 1D" {
          n301 = call-poly "V2D_Poly.vi"("Variant"=w660) -> ("Bool 1D"=w662:bool[])  [unwired: 10 in]
          n302 = Reverse 1D Array(array=w662) -> (reversed array=w661:bool[])
          n303 = To Variant(anything=w661) -> (Variant=w659:variant)
        }
      }
      n304 = call-dynamic "Add RTV.vi"("RT Variables in"=w650, "RTV name"=w645, "Data"=w644, "Scope"=w646, "error in (no error)"=w649) -> ("error out"=w643:errorcluster)  [unwired: 9 in, 1 out]
    }
    frame "range by start stop" {
      n305 = call "Var to String.vi"("Variant"=w671) -> ()  [unwired: 10 in, 1 out]
      n306 = Subtract(x=w668, y=w664) -> (x-y=w667:i32)
      n307 = Increment(x=w667) -> (x+1=w666:i32)
      n308 = for {
        N: w666 -> [_]
        tunnel: [w672] -> w665 mode=indexing
        i -> [w672]
      }
      n309 = Add(x=w665, y=w664) -> (x+y=w663:i32[])
      n310 = To Variant(anything=w663) -> (Variant=w670:variant)
    }
    frame "range by start stop step" {
      n311 = call "Var to String.vi"("Variant"=w684) -> ()  [unwired: 10 in, 1 out]
      n312 = Subtract(x=w681, y=w679) -> (x-y=w680:i32)
      n313 = Increment(x=w680) -> (x+1=w678:i32)
      n314 = Quotient & Remainder(x=w678, y=w675) -> (floor(x/y)=w677:i32)  [unwired: 1 out]
      n315 = for {
        N: w677 -> [_]
        tunnel: [w685] -> w674 mode=indexing
        i -> [w685]
      }
      n316 = Multiply(x=w675, y=w674) -> (x*y=w673:i32[])
      n317 = Add(x=w673, y=w679) -> (x+y=w676:i32[])
      n318 = To Variant(anything=w676) -> (Variant=w683:variant)
    }
  }
  "Return" <- w14
  n319 = Merge Errors(w18) -> (→"error out":errorcluster)
